vi "Filter by Action.vi"(10 "Action":string, 11 "Chronological List in":refnum<class "Chronological List.lvclass">) -> (2 "Include?":bool, 3 "Chronological List out":refnum<class "Chronological List.lvclass">)   [LabVIEW 2020, in "Chronological List.lvclass"]
uses:
  Chronological List.lvclass
  Chronological List.lvclass/Chronological List.ctl
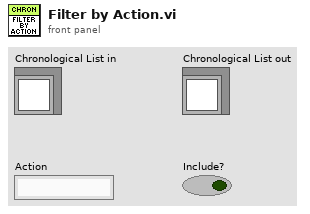
[diagram p1: front panel]
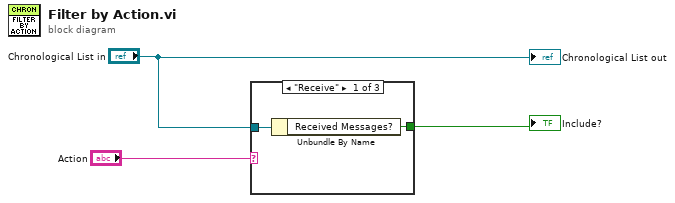
[diagram p0: block diagram]
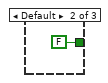
[diagram p2: hidden frame]
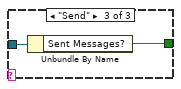
[diagram p3: hidden frame]
diagram:
  n1 = case shown="\"Receive\"" "Action" {
    tunnel: "Chronological List in" -> [w5 _ w8]
    tunnel: [w4 FALSE ("Sent Messages?") w7] -> w3
    frame "Receive" {
      n2 = Unbundle By Name(w5) -> ("Received Messages?"=w4:bool)
    }
    frame Default {
    }
    frame "Send" {
      n3 = Unbundle By Name(w8) -> ("Sent Messages?"=w7:bool)
    }
  }
  "Include?" <- w3
  "Chronological List out" <- "Chronological List in"
